vi "SMO.jsonRPC.DecodeResponse.vi"(7 "result type":variant, 8 "error in (no error)":errorcluster, 11 "jsonRPC response":refnum<class "Response.lvclass">) -> (0 "error out":errorcluster, 1 "id":i32, 3 "result":variant)   [LabVIEW 2013, in "SMO.jsonRPC.lvclass"]
doc: "---------------------------------------------------------------\nJKI State Machine Objects™\nhttp://jki.net/state-machine-objects/\nCopyright (C) 2005-2015, JKI <info@jki.net>\nALL RIGHTS RESERVEDJKI State Machine Objects (SMO) 1.0.0.5\nJKI - JKI\nCopyright (c) 2016, JKI"
uses:
  SMO.jsonRPC.lvclass
  <vilib>/JKI/JKI JSON RPC Specification/Response/Response.lvclass
  <vilib>/JKI/JKI JSON RPC Specification/Response/Response.lvclass/Response.ctl
  <vilib>/Utility/VariantDataType/GetTypeInfo.vi
  <vilib>/JKI/JKI JSON RPC Specification/Error/Error.lvclass
panel:
  # "For instructions on how to use the JKI State Machine Objects, examples and video tutorials, visit:\nhttp://jki.net/state-machine-objects/\n\nJKI State Machine Objects™\nhttp://jki.net/state-machine-objects/\nCopyright (C) 2005-2015, JKI <info@jki.net>\nALL RIGHTS RESERVED"
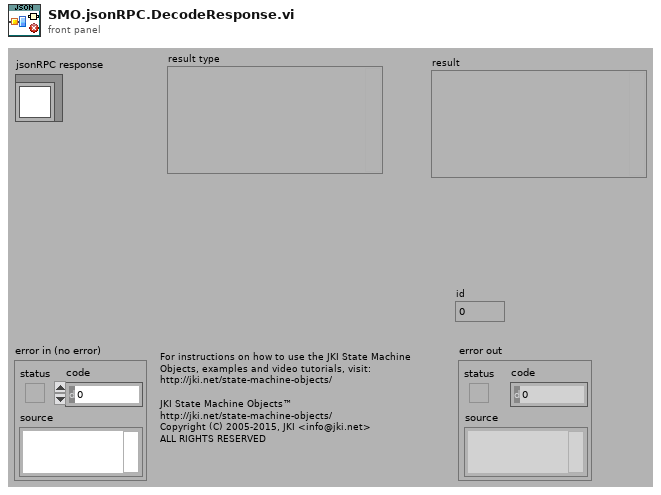
[diagram p1: front panel]
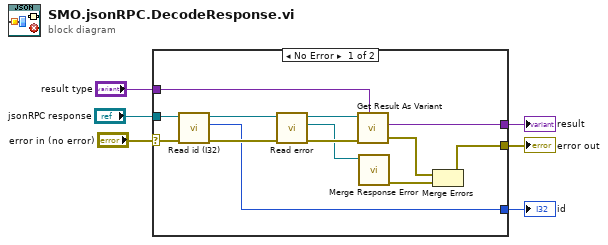
[diagram p0: block diagram]
diagram:
  n1 = case shown="No Error" "error in (no error)" {
    selector: "error in (no error)" -> [w9 w21]
    tunnel: [w14 w21] -> w6
    tunnel: "jsonRPC response" -> [w11 _]
    tunnel: "result type" -> [w19 w20]
    tunnel: [w18 w20] -> w2
    tunnel: [w7 _] -> w1
    frame No Error {
      n2 = call <vilib>:"Read id (I32).vi"("error in (no error)"=w9, "Response in"=w11) -> ("error out"=w8:errorcluster, "id"=w7:i32, "Response out"=w10:refnum<class "Response.lvclass">)  [unwired: 7 in]
      n3 = call <vilib>:"Read error.vi"("error in (no error)"=w8, "Response in"=w10) -> ("error out"=w16:errorcluster, "Error"=w13:refnum<class "Error.lvclass">, "Response out"=w17:refnum<class "Response.lvclass">)  [unwired: 7 in]
      n4 = call <vilib>:"Get Result As Variant.vi"("type"=w19, "error in (no error)"=w16, "Response in"=w17) -> ("error out"=w15:errorcluster, "result"=w18:variant)  [unwired: 6 in, 1 out]
      n5 = call <vilib>:"Merge Response Error.vi"("Error in"=w13) -> ("error out"=w12:errorcluster)  [unwired: 9 in, 1 out]
      n6 = Merge Errors(w15, w12) -> (w14:errorcluster)
    }
    frame Error {
    }
  }
  "error out" <- w6
  "result" <- w2
  "id" <- w1
